vi "Facto.vi"(1 "Factoriel souhaité":i32) -> (0 "Résultat":i32)   [LabVIEW 2018]
panel:
  out "Indice de boucle":i32
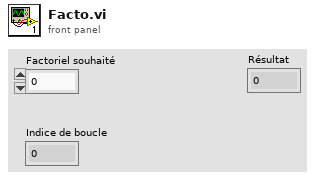
[diagram p1: front panel]
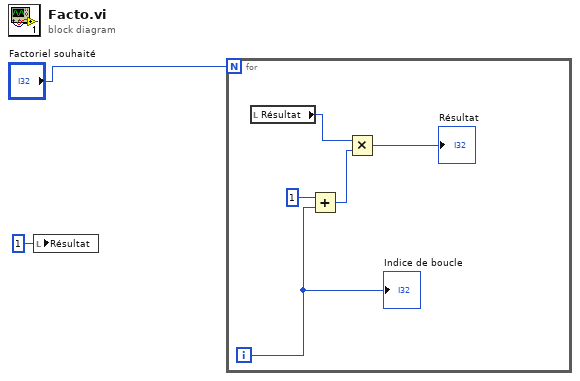
[diagram p0: block diagram]
diagram:
  n1 = local write "Résultat"(1 ("Résultat")) -> ()
  n2 = for {
    N: "Factoriel souhaité" -> [_]
    i -> [w5]
    n3 = local read "Résultat"() -> (w7:i32)
    n4 = Add(x=1, y=w5) -> (x+y=w4:i32)
    n5 = Multiply(x=w7, y=w4) -> (x*y=→"Résultat":i32)
    "Indice de boucle" <- w5
  }
